vi "LCR_Readout.vi"(8 "error in (no error)":errorcluster, 10 "Frequency in Hz":i32, 11 "WK6425 in":refnum<class "WK6425.lvclass">) -> (0 "error out":errorcluster, 1 "Resistance in Ohm":dbl, 2 "Capacitance in pF":dbl, 3 "WK6425 out":refnum<class "WK6425.lvclass">)   [LabVIEW 2013, in "WK6425.lvclass"]
uses:
  WK6425.lvclass
  InstrControl.lvclass
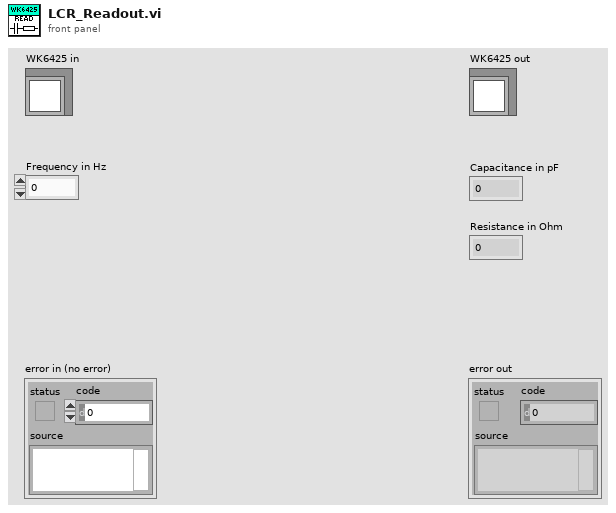
[diagram p1: front panel]
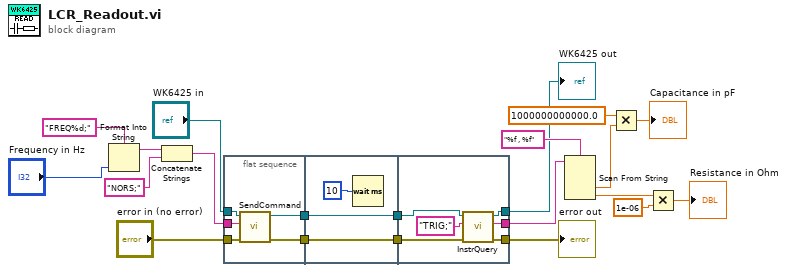
[diagram p0: block diagram]
diagram:
  n1 = Format Into String(format string="FREQ%d;", "Frequency in Hz") -> (resulting string=w15:string)  [unwired: 2 in, 1 out]
  n2 = Concatenate Strings(w15, "NORS;") -> (w16:string)
  n3 = flat-sequence {
    tunnel: w16 -> [w24]
    tunnel: "error in (no error)" -> [w26]
    tunnel: "WK6425 in" -> [w22]
    tunnel: [w25] -> w20
    tunnel: [w23] -> w19
    tunnel: w20 -> [w28]
    tunnel: [w28] -> w18
    tunnel: w19 -> [w27]
    tunnel: [w27] -> w17
    tunnel: [w34] -> w5
    tunnel: [w33] -> w9
    tunnel: w18 -> [w35]
    tunnel: w17 -> [w31]
    tunnel: [w30] -> w6
    frame #0 {
      n4 = call "SendCommand.vi"("error in (no error)"=w26, "Command string"=w24, "InstControl in"=w22) -> ("error out"=w25:errorcluster, "InstControl out"=w23:refnum<class "WK6425.lvclass">)  [unwired: 7 in]
    }
    frame #1 {
      n5 = Wait (ms)(milliseconds to wait=10) -> ()  [unwired: 1 out]
    }
    frame #2 {
      n6 = call-dynamic "InstrQuery.vi"("error in (no error)"=w35, "Command string"="TRIG;", "InstControl in"=w31) -> ("error out"=w34:errorcluster, "Instrument response"=w33:string, "InstControl out"=w30:refnum<class "WK6425.lvclass">)  [unwired: 6 in]
    }
  }
  n7 = Scan From String(format string="%f , %f", input string=w9) -> (output 1=w10:dbl, output 2=w2:dbl)  [unwired: 4 in, 3 out]
  n8 = Multiply(x=1000000000000.0 ("y"), y=w10) -> (x*y=→"Capacitance in pF":dbl)
  n9 = Multiply(x=w2, y=1e-06) -> (x*y=→"Resistance in Ohm":dbl)
  "error out" <- w5
  "WK6425 out" <- w6
